vi "02Manejo_panel 492.vi"(0 "Config Equipos":T2(array[cluster]) {"Ref PD" max=10000 step=1; "Med Princ" items=["1", "2", "3", "4", "5", "6", "7", "8", "9", "10", "11", "12", "13", "14", "15", "16", "17", "18", "19", "20", "21", "22", "23", "24", "25", "26", "27", "28", "29", "30", "31", "32"]}, 1 "Med nº":u8, 2 "Mediciones":T1, 3 "Nº equipo":i32, 4 "Paneles in":T4(array[cluster]) {"Nº" min=1.0 max=60.0 step=1.0 format="%#2.1f"; "Ultima recepción" format="%<%d/%m - %X>T"; "Med\nPpal" format="%_4g"}) -> (5 "Paneles out":T3(array[cluster]) {"Numeric" min=1.0 max=60.0 step=1.0 format="%#2.1f"; "Ultima recepción" format="%<%d/%m - %X>T"; "Med\nPpal" format="%_4g"})   [LabVIEW 2010]
panel:
  in  "Flags recep":bool[](array[boolean])
  out "T. error":timestamp[](array[timestamp])
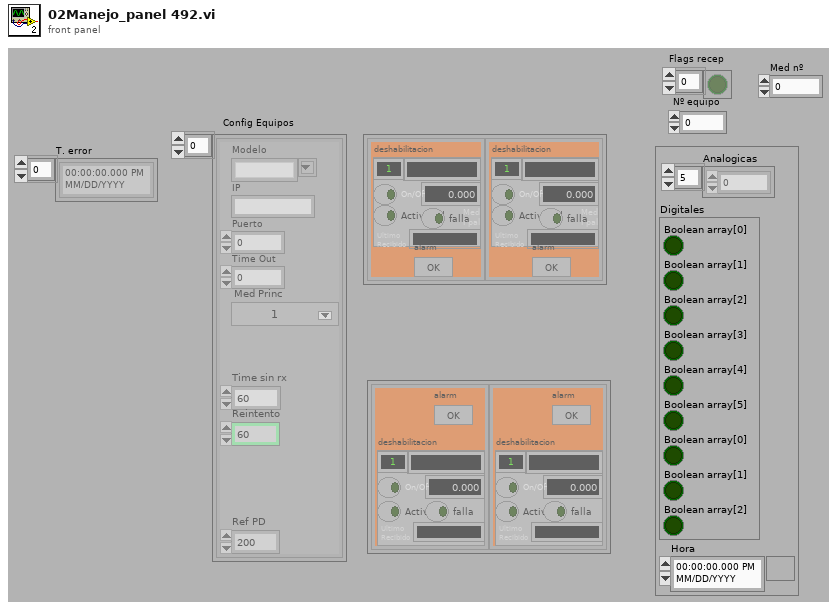
[diagram p1: front panel]
types:
  T1 = cluster{"Analogicas":sgl[], "Digitales":cluster{"Boolean array[0]":bool, "Boolean array[1]":bool, "Boolean array[2]":bool, "Boolean array[3]":bool, "Boolean array[4]":bool, "Boolean array[5]":bool, "Boolean array[0]":bool, "Boolean array[1]":bool, "Boolean array[2]":bool}, "Hora":timestamp}
  T2 = cluster{"Modelo":string, "IP":string, "Puerto":u16, "Time Out":u16, "Med Princ":u16, "Time sin rx":u16, "Reintento":u16, "Ref PD":u16}[]
  T3 = cluster{"Nombre":string, "Med\nPpal":dbl, "On/Off":bool, "Ultima recepción":timestamp, "Numeric":dbl, "deshabilitacion":bool, "Actividad":bool, "falla":bool, "alarm":bool}[][]
  T4 = cluster{"Nombre":string, "Med\nPpal":dbl, "On/Off":bool, "Ultima recepción":timestamp, "Nº":dbl, "deshabilitacion":bool, "Actividad":bool, "falla":bool, "alarm":bool}[][]
  T5 = cluster{"Boolean array[0]":bool, "Boolean array[1]":bool, "Boolean array[2]":bool, "Boolean array[3]":bool, "Boolean array[4]":bool, "Boolean array[5]":bool, "Boolean array[0]":bool, "Boolean array[1]":bool, "Boolean array[2]":bool}
  T6 = cluster{"Modelo":string, "IP":string, "Puerto":u16, "Time Out":u16, "Med Princ":u16, "Time sin rx":u16, "Reintento":u16, "Ref PD":u16}
  T7 = cluster{bool, bool, bool, bool, bool, bool, bool, bool, bool, bool}
  T8 = cluster{"Nombre":string, "Med\nPpal":dbl, "On/Off":bool, "Ultima recepción":timestamp, "Nº":dbl, "deshabilitacion":bool, "Actividad":bool, "falla":bool, "alarm":bool}
  T9 = cluster{"Nombre":string, "Numeric":sgl, "On/Off":bool, "Ultima recepción":timestamp, "Nº":dbl, "deshabilitacion":bool, bool, bool, bool}
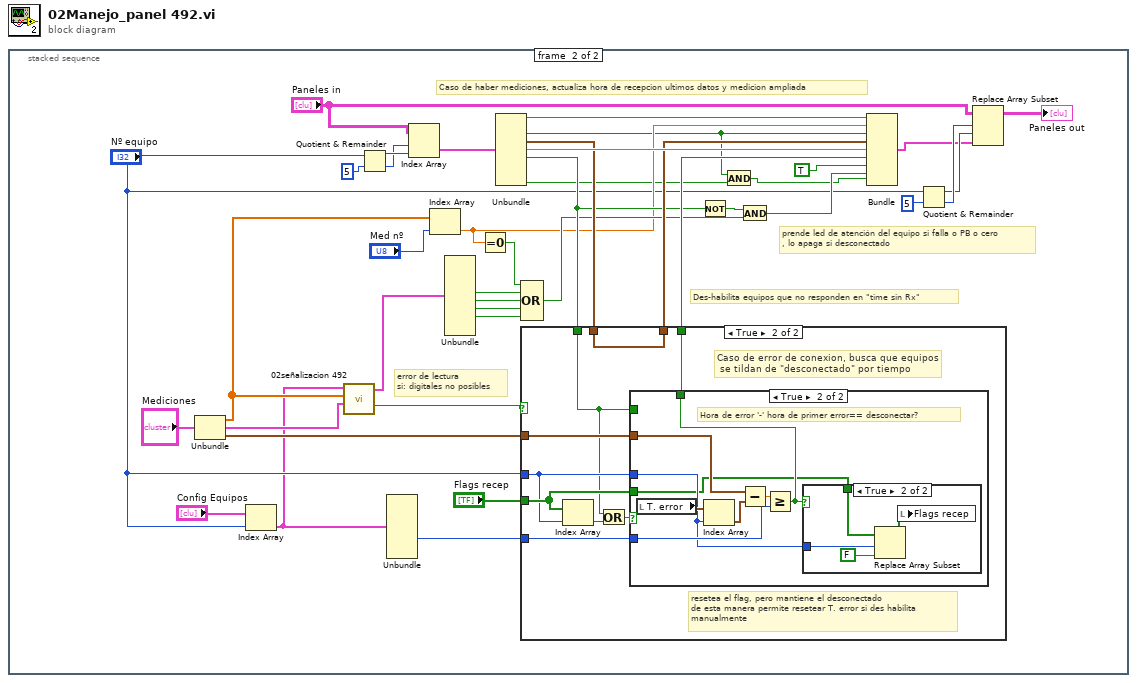
[diagram p0: block diagram]
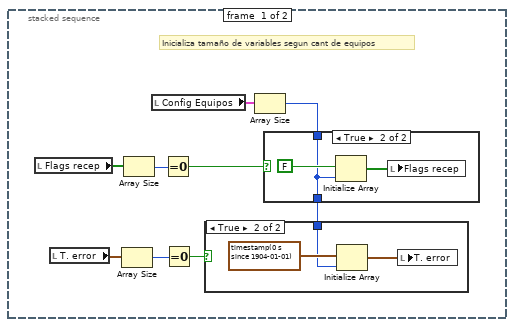
[diagram p2: hidden frame]
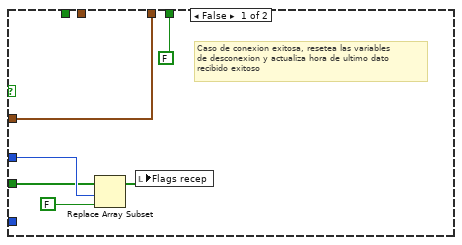
[diagram p5: hidden frame]
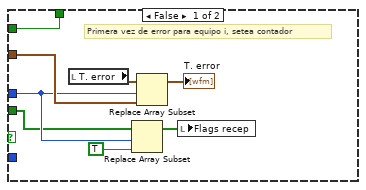
[diagram p6: hidden frame]
diagram:
  n1 = stacked-sequence {
    frame #0 {
      # "Inicializa tamaño de variables segun cant de equipos"
      n2 = local read "Flags recep"() -> (w9:bool[])
      n3 = local read "T. error"() -> (w8:timestamp[])
      n4 = Array Size(array=w8) -> (size(s)=w4:i32)
      n5 = Array Size(array=w9) -> (size(s)=w7:i32)
      n6 = local read "Config Equipos"() -> (w3:T2)
      n7 = Equal To 0?(x=w7) -> (x = 0?=w6:bool)
      n8 = Equal To 0?(x=w4) -> (x = 0?=w5:bool)
      n9 = Array Size(array=w3) -> (size(s)=w2:i32)
      n10 = case shown="True" w6 {
        tunnel: w2 -> [w13 w14]
        tunnel: [w13 w14] -> w1
        frame False {
        }
        frame True {
          n11 = Initialize Array(FALSE, w14) -> (w16:bool[])
          n12 = local write "Flags recep"(w16) -> ()
        }
      }
      n13 = case shown="True" w5 {
        tunnel: w1 -> [_ w10]
        frame False {
        }
        frame True {
          n14 = Initialize Array(timestamp(0 s since 1904-01-01), w10) -> (w12:timestamp[])
          n15 = local write "T. error"(w12) -> ()
        }
      }
    }
    frame #1 {
      # "error de lectura\nsi: digitales no posibles"
      # "prende led de atención del equipo si falla o PB o cero\n, lo apaga si desconectado"
      # "Des-habilita equipos que no responden en \"time sin Rx\""
      # "Caso de haber mediciones, actualiza hora de recepcion ultimos datos y medicion ampliada"
      n16 = Unbundle("Mediciones") -> ("Analogicas"=w18:sgl[], "Digitales"=w19:T5, "Hora"=w49:timestamp)
      n17 = Index Array(array="Config Equipos", index="Nº equipo") -> (element=w17:T6)
      n18 = call "02señalizacion 492.vi"("Digitales"=w19, "Analogicas"=w18, "Config Equipo"=w17) -> ("Error Logico"=w20:bool, "Señalizacion"=w21:T7)  [unwired: 3 in]
      n19 = Quotient & Remainder(x="Nº equipo", y=5) -> (x-y*floor(x/y)=w30:i32, floor(x/y)=w29:i32)
      n20 = Unbundle(w17) -> ("Time sin rx"=w50:u16)  [unwired: 7 out]
      n21 = Index Array(array="Paneles in", index (row)=w29, index (col)=w30) -> (element=w28:T8)
      n22 = Index Array(array=w18, index="Med nº") -> (element=w40:sgl)
      n23 = Unbundle(w21) -> (w45:bool, w46:bool, w47:bool, w48:bool)  [unwired: 6 out]
      n24 = Equal To 0?(x=w40) -> (x = 0?=w39:bool)
      n25 = Unbundle(w28) -> ("Nombre"=w56:string, "On/Off"=w24:bool, "Ultima recepción"=w54:timestamp, "Nº"=w57:dbl, "deshabilitacion"=w44:bool, "alarm"=w23:bool)  [unwired: 3 out]
      n26 = Compound Arithmetic op=OR(w39, w45, w46, w47, w48) -> (w41:bool)
      n27 = case shown="True" w20 {
        tunnel: w49 -> [w63 w71]
        tunnel: [w63 w72] -> w55
        tunnel: w54 -> [_ w72]
        tunnel: w50 -> [_ w70]
        tunnel: "Nº equipo" -> [w60 w68]
        tunnel: "Flags recep" -> [w59 w69]
        tunnel: w44 -> [_ w64]
        tunnel: [FALSE ("new element/subarray") w66] -> w52
        frame False {
          # "Caso de conexion exitosa, resetea las variables\nde desconexion y actualiza hora de ultimo dato\nrecibido exitoso"
          n28 = Replace Array Subset(array=w59, new element=FALSE ("new element/subarray"), index=w60) -> (w62:bool[])
          n29 = local write "Flags recep"(w62) -> ()
        }
        frame True {
          # "resetea el flag, pero mantiene el desconectado\nde esta manera permite resetear T. error si des habilita\nmanualmente"
          # "Caso de error de conexion, busca que equipos\n se tildan de \"desconectado\" por tiempo"
          n30 = Index Array(array=w69, index=w68) -> (element=w65:bool)
          n31 = Or(x=w64, y=w65) -> (x .or. y?=w67:bool)
          n32 = case shown="True" w67 {
            tunnel: w71 -> [w76 w88]
            tunnel: w70 -> [_ w84]
            tunnel: w68 -> [w75 w83]
            tunnel: w69 -> [w74 w81]
            tunnel: w64 -> [w73 _]
            tunnel: [w73 w82] -> w66
            frame False {
              # "Primera vez de error para equipo i, setea contador"
              n33 = local read "T. error"() -> (w80:timestamp[])
              n34 = Replace Array Subset(array=w74, new element=TRUE ("new element/subarray"), index=w75) -> (w78:bool[])
              n35 = Replace Array Subset(array=w80, new element=w76, index=w75) -> (→"T. error":timestamp[])
              n36 = local write "Flags recep"(w78) -> ()
            }
            frame True {
              # "Hora de error '-' hora de primer error== desconectar?"
              n37 = local read "T. error"() -> (w87:timestamp[])
              n38 = Index Array(array=w87, index=w83) -> (element=w86:timestamp)
              n39 = Subtract(x=w88, y=w86) -> (x-y=w85:dbl)
              n40 = Greater Or Equal?(x=w85, y=w84) -> (x >= y?=w82:bool)
              n41 = case shown="True" w82 {
                tunnel: w83 -> [_ w91]
                tunnel: w81 -> [_ w89]
                frame False {
                }
                frame True {
                  n42 = Replace Array Subset(array=w89, new element=FALSE ("new element/subarray"), index=w91) -> (w92:bool[])
                  n43 = local write "Flags recep"(w92) -> ()
                }
              }
            }
          }
        }
      }
      n44 = Not(x=w44) -> (.not. x?=w42:bool)
      n45 = And(x=w24, y=w23) -> (x .and. y?=w25:bool)
      n46 = And(x=w42, y=w41) -> (x .and. y?=w43:bool)
      n47 = Bundle("Nombre"=w56, "Numeric"=w40, "On/Off"=w24, "Ultima recepción"=w55, "Nº"=w57, "deshabilitacion"=w52, TRUE, w43, w25) -> (w32:T9)  [unwired: 1 out]
      n48 = Quotient & Remainder(x="Nº equipo", y=5) -> (x-y*floor(x/y)=w35:i32, floor(x/y)=w36:i32)
      n49 = Replace Array Subset(array="Paneles in", new element=w32, index (row)=w36, index (col)=w35) -> (→"Paneles out":T4)
    }
  }
